vi "Set Account Information.vi"(8 "error in (no error)":errorcluster, 11 "Bank Account in":refnum<class "Bank Account.lvclass">) -> (0 "error out":errorcluster, 3 "Bank Account out":refnum<class "Bank Account.lvclass">)   [LabVIEW 2016, in "CLD Exam - ATM.lvlib" / "Bank Account.lvclass"]
uses:
  Bank Account.lvclass
  Bank Account.lvclass/Bank Account.ctl
  <vilib>/Utility/file.llb/Read Delimited Spreadsheet (string).vi
  <vilib>/Utility/file.llb/Write Delimited Spreadsheet (string).vi
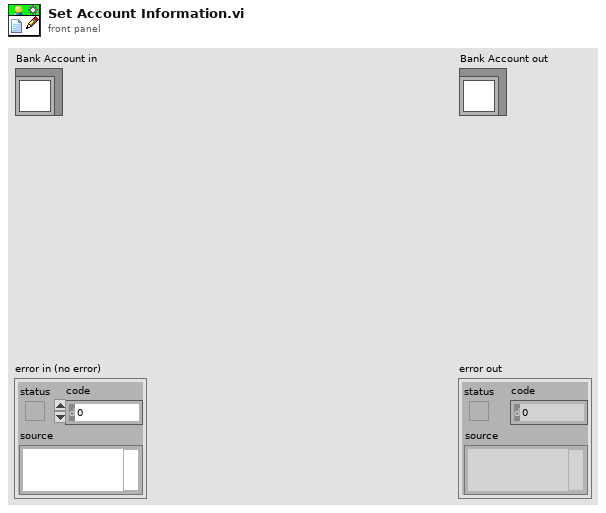
[diagram p1: front panel]
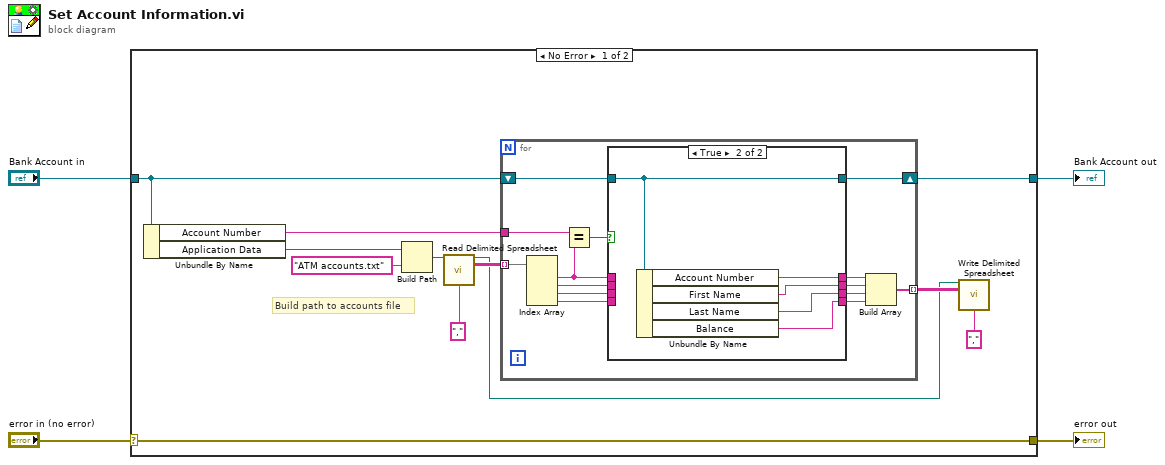
[diagram p0: block diagram]
diagram:
  n1 = case shown="No Error" "error in (no error)" {
    selector: "error in (no error)" -> [w16 w42]
    tunnel: [w16 w42] -> w3
    tunnel: [w10 w41] -> w1
    tunnel: "Bank Account in" -> [w11 w41]
    frame No Error {
      # "Build path to accounts file"
      n2 = Unbundle By Name(w11) -> ("Account Number"=w8:string, "Application Data"=w9:path)
      n3 = Build Path(base path=w9, name or relative path="ATM accounts.txt") -> (appended path=w14:path)
      n4 = call-poly <vilib>:"Read Delimited Spreadsheet.vi"("file path (dialog if empty)"=w14, "delimiter (\\t)"="," ("delimiter (\\t)")) -> ("new file path (Not A Path if cancelled)"=w6:path, "all rows"=w12:string[][])  [unwired: 8 in, 4 out]
      n5 = for {
        tunnel: w12 -> [w30] mode=indexing
        tunnel: w8 -> [w29]
        shift-right: [w22] -> w10
        shift-left: w11 -> [w23]
        tunnel: [w17] -> w7 mode=indexing
        n6 = Index Array(array=w30) -> (element #1=w27:string, element #2=w26:string, element #3=w25:string, element #4=w24:string)  [unwired: 4 in]
        n7 = Equal?(x=w29, y=w27) -> (x = y?=w28:bool)
        n8 = case shown="True" w28 {
          tunnel: w27 -> [w35 _]
          tunnel: w26 -> [w34 _]
          tunnel: w25 -> [w33 _]
          tunnel: w24 -> [w32 _]
          tunnel: [w35 w39] -> w21
          tunnel: [w34 w38] -> w20
          tunnel: [w33 w37] -> w19
          tunnel: [w32 w36] -> w18
          tunnel: [w31 w40] -> w22
          tunnel: w23 -> [w31 w40]
          frame False {
          }
          frame True {
            n9 = Unbundle By Name(w40) -> ("Account Number"=w39:string, "First Name"=w38:string, "Last Name"=w37:string, "Balance"=w36:string)
          }
        }
        n10 = Build Array(w21, w20, w19, w18) -> (w17:string[])
      }
      n11 = call-poly <vilib>:"Write Delimited Spreadsheet.vi"("file path (dialog if empty)"=w6, "2D data"=w7, "delimiter (\\t)"="," ("delimiter (\\t)")) -> ()  [unwired: 11 in, 2 out]
    }
    frame Error {
    }
  }
  "error out" <- w3
  "Bank Account out" <- w1
